vi "Point&Path@Swap__Parameter.vi"(1 "ParamterIn":string) -> (0 "ParamterOut":string)   [LabVIEW 2019]
panel:
  in  "Axis 7":string(combo)="H"
  in  "Axis 6":string(combo)="0"
  in  "Axis 5":string(combo)="0"
  in  "Axis 4":string(combo)="0"
  in  "Axis 3":string(combo)="Z"
  in  "Axis 2":string(combo)="Y"
  out "PointNameList":string[](array[string])
  in  "Axis 1":string(combo)="X"
  in  "PointName":string(combo)
  in  "Confirm":bool
  # "Point&Path@Swap $Point,&&&&&&&\n&= X Y Z U V W H 0\nExample: Point, YXZUVWH will change XY only"
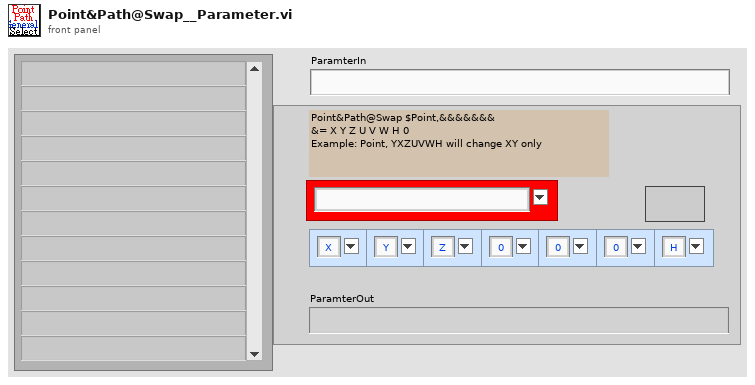
[diagram p1: front panel]
types:
  T1 = enum16{"Get", "UpdatePointS", "Init", "UpdateIndex", "GetCurrent&Index+1", "GetWithIndex", "ChkLast", "GetCurrent"}
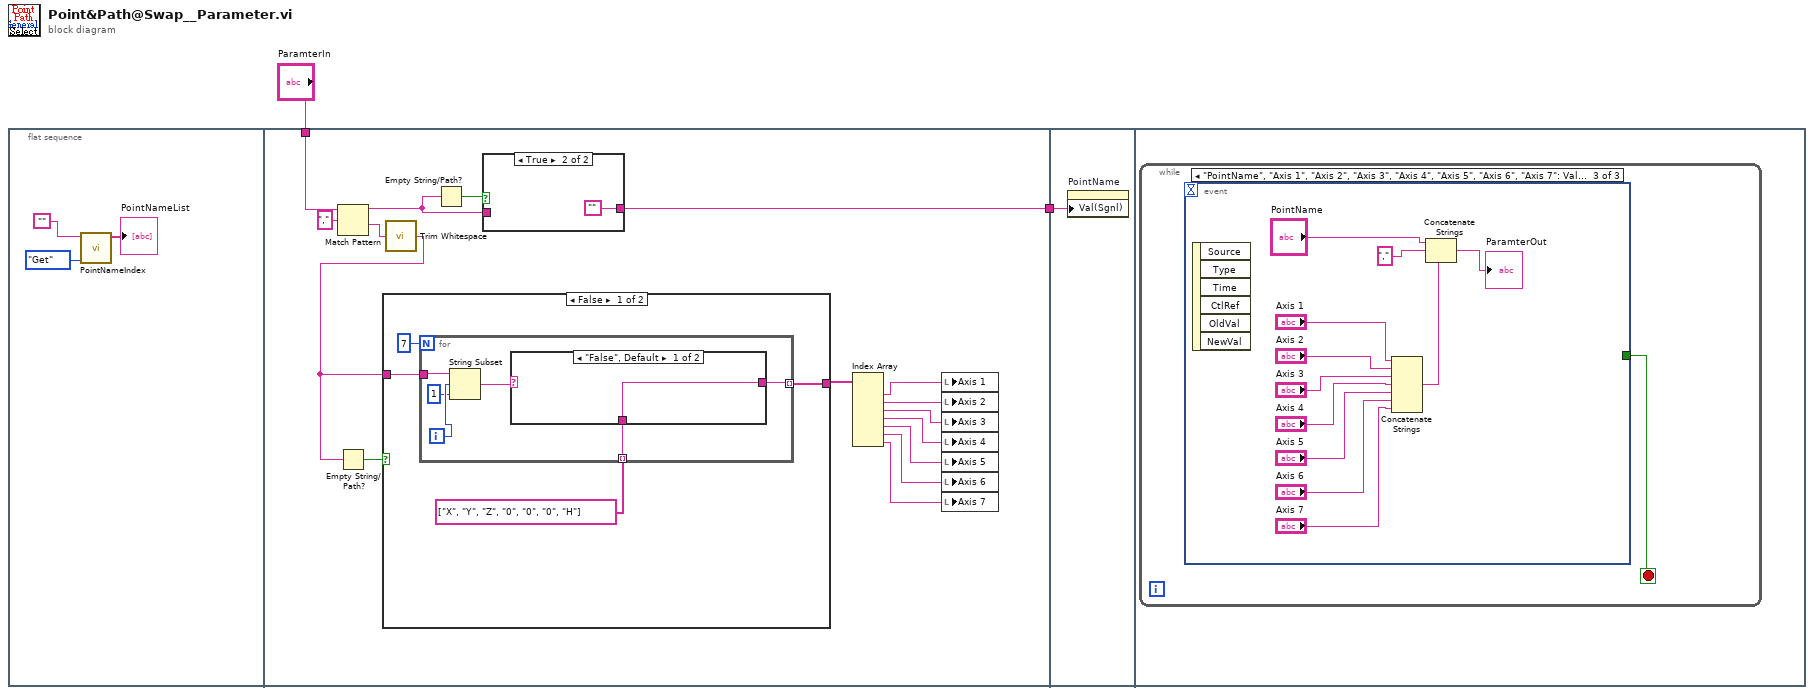
[diagram p0: block diagram]
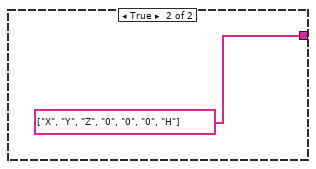
[diagram p3: hidden frame]
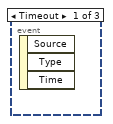
[diagram p5: hidden frame]
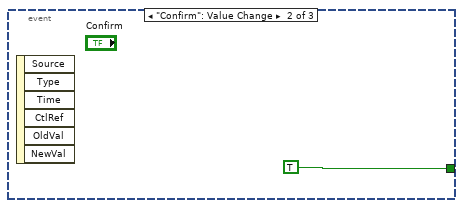
[diagram p6: hidden frame]
diagram:
  n1 = flat-sequence {
    tunnel: "ParamterIn" -> [w20]
    tunnel: [w17] -> w1
    tunnel: w1 -> [w37]
    frame #0 {
      n2 = call "PointNameIndex.vi"("OP"=T1."Get", "PointName"="") -> ("PointNameList"=→"PointNameList":string[])  [unwired: 4 in, 5 out]
    }
    frame #1 {
      n3 = Match Pattern(string=w20, regular expression="," ("search string")) -> (before substring=w18:string, after substring=w16:string)  [unwired: 1 in, 2 out]
      n4 = call <vilib>:"Trim Whitespace.vi"("string"=w16) -> ("trimmed string"=w14:string)  [unwired: 1 in]
      n5 = Empty String/Path?(string/path=w14) -> (empty?=w15:bool)
      n6 = case shown="False" w15 {
        tunnel: w14 -> [w24 _]
        tunnel: [w22 string[] ["X", "Y", "Z", "0", "0", "0", "H"] ("Array")] -> w13
        frame False {
          n7 = for {
            N: 7 -> [_]
            tunnel: w24 -> [w31]
            tunnel: [w27] -> w22 mode=indexing
            tunnel: string[] ["X", "Y", "Z", "0", "0", "0", "H"] ("Array") -> [w26] mode=indexing
            i -> [w30]
            n8 = String Subset(string=w31, offset (0)=w30, length (rest)=1 ("length (rest)")) -> (substring=w28:string)
            n9 = case shown="\"False\", Default" w28 {
              selector: w28 -> [_ w33]
              tunnel: [w32 w33] -> w27
              tunnel: w26 -> [w32 _]
              frame "False", Default {
              }
              frame "0", "H", "U", "V", "W", "X", "Y", "Z" {
              }
            }
          }
        }
        frame True {
        }
      }
      n10 = Empty String/Path?(string/path=w18) -> (empty?=w21:bool)
      n11 = case shown="True" w21 {
        tunnel: w18 -> [w35 _]
        tunnel: [w35 ""] -> w17
        frame False {
        }
        frame True {
        }
      }
      n12 = Index Array(array=w13) -> (element #1=w12:string, element #2=w11:string, element #3=w10:string, element #4=w9:string, element #5=w8:string, element #6=w7:string, element #7=w6:string)  [unwired: 7 in]
      n13 = local write "Axis 1"(w12) -> ()
      n14 = local write "Axis 2"(w11) -> ()
      n15 = local write "Axis 3"(w10) -> ()
      n16 = local write "Axis 4"(w9) -> ()
      n17 = local write "Axis 5"(w8) -> ()
      n18 = local write "Axis 6"(w7) -> ()
      n19 = local write "Axis 7"(w6) -> ()
    }
    frame #2 {
      n20 = property on="PointName" class="CmbBox"("Val(Sgnl)"=w37) -> ()  [unwired: 2 in, 2 out]
    }
    frame #3 {
      n21 = while {
        stop <- w38 stop-if-true
        n22 = event shown="[2] \"PointName\", \"Axis 1\", \"Axis 2\", \"Axis 3\", \"Axis 4\", \"Axis 5\", \"Axis 6\", \"Axis 7\": Value Change" {
          selector: _ -> [_ _ _]
          dyn-events: _ -> [_ _ _]
          timeout: _ -> [_ _ _]
          tunnel: [_ TRUE _] -> w38
          event Timeout {
            n23 = event-data() -> ()  [unwired: 1 in, 3 out]
          }
          event "Confirm": Value Change {
            n24 = event-data() -> ()  [unwired: 1 in, 6 out]
          }
          event "PointName", "Axis 1", "Axis 2", "Axis 3", "Axis 4", "Axis 5", "Axis 6", "Axis 7": Value Change {
            n25 = event-data() -> ()  [unwired: 1 in, 6 out]
            n26 = Concatenate Strings("Axis 1", "Axis 2", "Axis 3", "Axis 4", "Axis 5", "Axis 6", "Axis 7") -> (w40:string)
            n27 = Concatenate Strings("PointName", ",", w40) -> (→"ParamterOut":string)
          }
        }
      }
    }
  }
